vi "get camera driver.vi"(8 "error in (no error)":errorcluster, 9 "Path":path, 10 "Section":string, 11 "SIM Thermal Camera Factory in":refnum<class "SIM Thermal Camera Factory.lvclass">) -> (0 "error out":errorcluster, 2 "Camera Driver.lvclass":refnum<class "Camera Driver.lvclass">)   [LabVIEW 2022 SP3, in "SIM Thermal Camera Factory.lvclass"]
uses:
  SIM Thermal Camera Factory.lvclass
  SIM Thermal Camera Factory.lvclass/SIM Thermal Camera Factory.ctl
  Sim Camera Driver/Sim Camera Driver.lvclass
  C:/XY Stage/XY Stage/Framework/Base/Base.lvclass
  C:/XY Stage/Camera/Sim Camera Driver/Sim Camera Driver.lvclass
  C:/XY Stage/Camera/Camera Driver/Camera Driver.lvclass
  Camera Driver/Camera Driver.lvclass
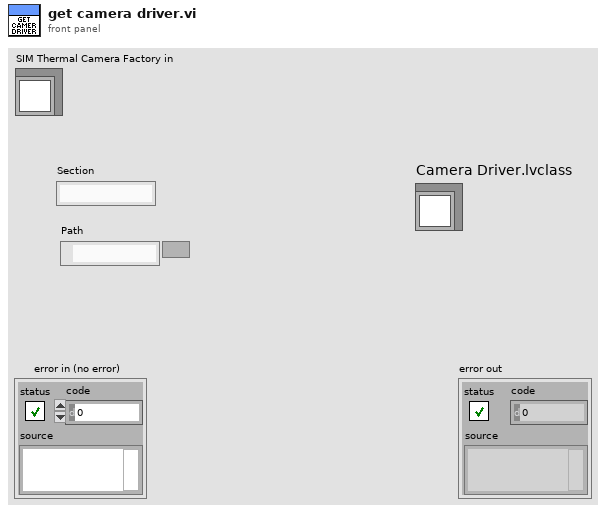
[diagram p1: front panel]
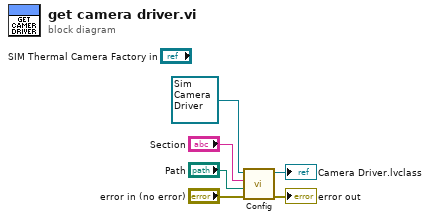
[diagram p0: block diagram]
diagram:
  n1 = call "Config.vi"("error in (no error)"="error in (no error)", "Path"="Path", "Section"="Section", "Sim Camera Driver in"=refnum<class "Sim Camera Driver.lvclass"> refnum ("Sim Camera Driver.lvclass")) -> ("error out"=→"error out":errorcluster, "Sim Camera Driver out"=→"Camera Driver.lvclass":refnum<class "Sim Camera Driver.lvclass">)  [unwired: 6 in]
